vi "standard executor.vi"(11 "task":refnum<class "task.lvclass">) -> ()   [LabVIEW 2013, in "thread pool.lvclass"]
uses:
  thread pool.lvclass
  task/task.lvclass
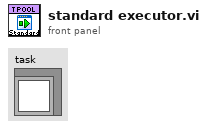
[diagram p1: front panel]
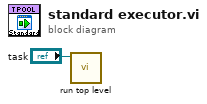
[diagram p0: block diagram]
diagram:
  n1 = call "run top level.vi"("task"="task") -> ()  [unwired: 11 in]
